vi "Fc_receiver_queue_Main_menu.vi"(8 "error in (no error)":errorcluster, 10 "Queue in":refnum<queue>, 11 "MulticolumnListbox in":refnum<vi>) -> (0 "error out":errorcluster, 3 "Queue out":refnum<queue>)   [LabVIEW 2021]
doc: "This function receives the data from the active windows and stores it in the queue to send in the main menu."
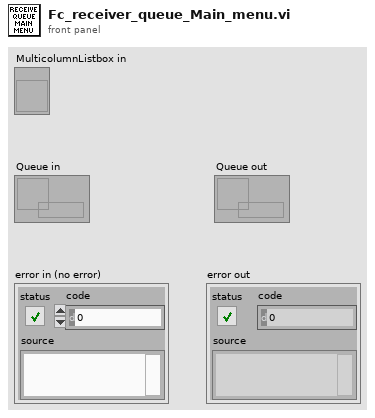
[diagram p1: front panel]
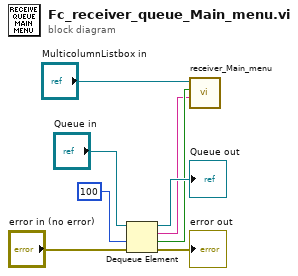
[diagram p0: block diagram]
diagram:
  n1 = Dequeue Element(queue="Queue in", timeout in ms (-1)=100, error in (no error)="error in (no error)") -> (queue out=→"Queue out":refnum<queue>, element=w2:string, timed out?=w3:bool, error out=→"error out":errorcluster)
  n2 = call "receiver_Main_menu.vi"("String"=w2, "timed out?"=w3, "MulticolumnListbox in"="MulticolumnListbox in") -> ()  [unwired: 9 in]
